vi "onProcessStarted.vi"(8 "error in (no error)":errorcluster, 11 "Instrument":refnum<class "Instrument.lvclass">) -> (0 "error out":errorcluster, 3 "Instrument out":refnum<class "Instrument.lvclass">)   [LabVIEW 2019, in "Instrument.lvclass"]
uses:
  Instrument.lvclass
  <vilib>/JKI/JKI SMO/SMO/SMO.lvclass
panel:
  # "For instructions on how to use the JKI State Machine Objects, examples and video tutorials, visit:\nhttp://jki.net/state-machine-objects/\n\nJKI State Machine Objects™\nhttp://jki.net/state-machine-objects/\nCopyright (C) 2005-2015, JKI <info@jki.net>\nALL RIGHTS RESERVED"
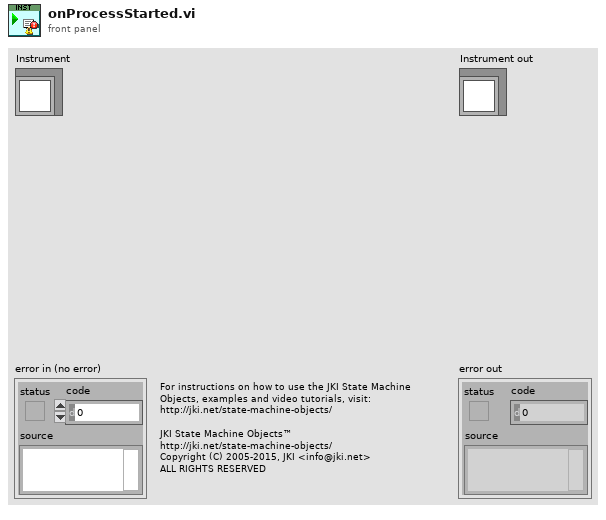
[diagram p1: front panel]
types:
  T1 = typedef "Instrument.lvclass/PrivateEvents--LogTime.ctl" = u32
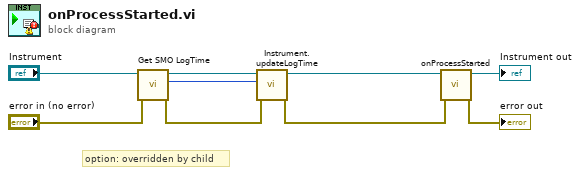
[diagram p0: block diagram]
diagram:
  # "option: overridden by child"
  n1 = call-dynamic "Get SMO LogTime.vi"("error in (no error)"="error in (no error)", "Instrument in"="Instrument") -> ("error out"=w1:errorcluster, "LogTime"=w3:T1, "Instrument out"=w4:refnum<class "Instrument.lvclass">)  [unwired: 7 in]
  n2 = call "Instrument.updateLogTime.vi"("error in (no error)"=w1, "LogTime"=w3, "Instrument"=w4) -> ("error out"=w6:errorcluster, "Instrument out"=w7:refnum<class "Instrument.lvclass">)  [unwired: 7 in]
  n3 = call-parent "onProcessStarted.vi"("error in (no error)"=w6, "SMO"=w7) -> ("error out"=→"error out":errorcluster, "SMO out"=→"Instrument out":refnum<class "Instrument.lvclass">)  [unwired: 8 in]
